vi "Teleop.vi"(10 "Match Info":T1={"Autonomous Elapsed Seconds"=0.0, "TeleOp Elapsed Seconds"=0.0, "Disabled Elapsed Seconds"=0.0, "Visited Autonomous"=FALSE, "Visited TeleOp"=FALSE, "Visited Disabled"=FALSE, "Autonomous Settings"={"Autonomous Style"=enum."Independent", "VI Refnum"=refnum}}, 11 "Call Context":T2) -> ()   [LabVIEW 2017]
doc: "This VI is called for each TeleOp packet received from the DS where the robot is not disabled. It is often used to read from the joysticks and update I/O or to update setpoints for timed control loops. It should complete and return within 20 milliseconds or it may miss DS packets."
uses:
  <vilib>/Rock Robotics/WPI/DriverStation/WPI_DriverStationDerivedRobotMode.ctl
  <vilib>/Rock Robotics/WPI/DriverStation/WPI_DriverStationMatch Info.ctl
  <vilib>/Rock Robotics/WPI/Utilities/WPI_GetSetVariantRefNum.vi
  <vilib>/Rock Robotics/WPI/RobotDrive/WPI_RobotDriveArcadeDrive_Standard(NoSaturation).vi
  Global Variables.vi
  <vilib>/Rock Robotics/Network Tables/NT Write Boolean Array.vi
  <vilib>/Rock Robotics/Network Tables/NT Write Numeric Array.vi
  <vilib>/Rock Robotics/Network Tables/NT Read Boolean.vi
  <vilib>/Rock Robotics/Network Tables/NT Read Number.vi
  <vilib>/Rock Robotics/WPI/RobotDrive/WPI_RobotDriveMecanumDrive_Cartesian.vi
panel:
  out "Sample Slider 0":dbl(slide) scale=0.0..5.0
  out "Sample Boolean 1":bool
  out "Sample Boolean 0":bool
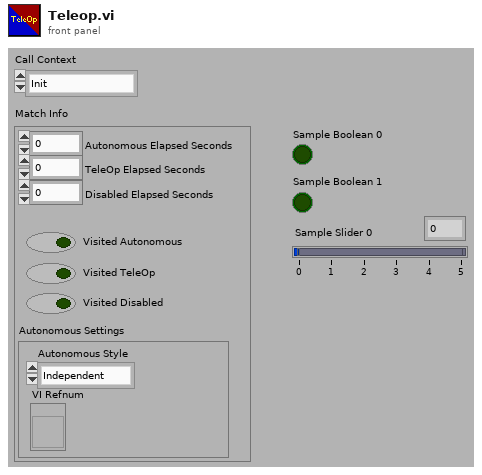
[diagram p1: front panel]
types:
  T1 = typedef "WPI_DriverStationMatch Info.ctl" = cluster{"Autonomous Elapsed Seconds":dbl, "TeleOp Elapsed Seconds":dbl, "Disabled Elapsed Seconds":dbl, "Visited Autonomous":bool, "Visited TeleOp":bool, "Visited Disabled":bool, "Autonomous Settings":cluster{"Autonomous Style":enum16{"Iterative", "Independent"}, "VI Refnum":refnum<vi>}}
  T2 = typedef "WPI_DriverStationDerivedRobotMode.ctl" = enum16{"Init", "Execute", "Stop"}
  T3 = typedef "WPI_RobotDriveDevRef.ctl" = cluster{"DevStatus":errorcluster, "Motors[]":T4[], "Square Inputs":bool, "Max Output":dbl}
  T4 = typedef "WPI_MotorControlDeviceRef.ctl" = cluster{"DeviceStatus":errorcluster, "Type":T5, "PWM":cluster{"PWM Channel":T6, "DeadBand":T7}, "CAN":cluster{"Device Number":u8, "SetOutput VI Ref":variant, "GetOutput VI Ref":variant, "Enable VI Ref":variant, "Disable VI Ref":variant, "Data":variant}, "Invert":bool, "DIO PWM":cluster{"PWM \"Enable\" Channel":T6, "DIOChannel":T8, "PWM Rate":dbl}}
  T5 = typedef "WPI_MotorControlType.ctl" = enum16{"PWM", "CAN", "DIO PWM"}
  T6 = typedef "FPGA_DIOPWMChannel.ctl" = enum8{"PWM 0", "PWM 1", "PWM 2", "PWM 3", "PWM 4", "PWM 5", "PWM 6", "PWM 7", "PWM 8", "PWM 9", "PWM MXP 0", "PWM MXP 1", "PWM MXP 2", "PWM MXP 3", "PWM MXP 4", "PWM MXP 5", "PWM MXP 6", "PWM MXP 7", "PWM MXP 8", "PWM MXP 9", "Invalid"}
  T7 = typedef "WPI_PWMDeadband.ctl" = cluster{"Name":string, "maxPositivePwm":i32, "minPositivePwm":i32, "centerPwm":i32, "maxNegativePwm":i32, "minNegativePwm":i32, "angularRange":u16}
  T8 = typedef "FPGA_DIOChannel.ctl" = enum8{"DIO 0", "DIO 1", "DIO 2", "DIO 3", "DIO 4", "DIO 5", "DIO 6", "DIO 7", "DIO 8", "DIO 9", "DIO MXP 0", "DIO MXP 1", "DIO MXP 2", "DIO MXP 3", "DIO MXP 4", "DIO MXP 5", "DIO MXP 6", "DIO MXP 7", "DIO MXP 8", "DIO MXP 9", "DIO MXP 10", "DIO MXP 11", "DIO MXP 12", "DIO MXP 13", "DIO MXP 14", "DIO MXP 15", "SPI Port CS1", "SPI Port CS2", "SPI Port CS3", "SPI Port MISO", "SPI Port MOSI", "Invalid"}
  T9 = typedef "WPI_JoystickDevRef.ctl" = cluster{"Device":T10}
  T10 = typedef "WPI_JoystickDeviceEnum.ctl" = enum16{"USB 0", "USB 1", "USB 2", "USB 3", "USB 4", "USB 5"}
  T11 = typedef "WPI_GyroDevRef.ctl" = cluster{"DevStatus":errorcluster, "Analog Channel":T12, "Gain (VoltsPerDegree/Second)":dbl, "Gyro Type":enum16{"Analog", "XRS450"}, "Handle":i32, "SPI Bus":T13, "Device Found":bool, "Sample Rate":dbl, "Calibrate On Open":bool, "Offset":dbl}
  T12 = typedef "FPGA_AIChannel.ctl" = enum8{"AI 0", "AI 1", "AI 2", "AI 3", "AI MXP 0", "AI MXP 1", "AI MXP 2", "AI MXP 3", "Invalid"}
  T13 = typedef "spi_bus.ctl" = enum16{"SPI On-Board, CS0", "SPI On-Board, CS1", "SPI On-Board, CS2", "SPI On-Board, CS3", "SPI MXP", "Invalid"}
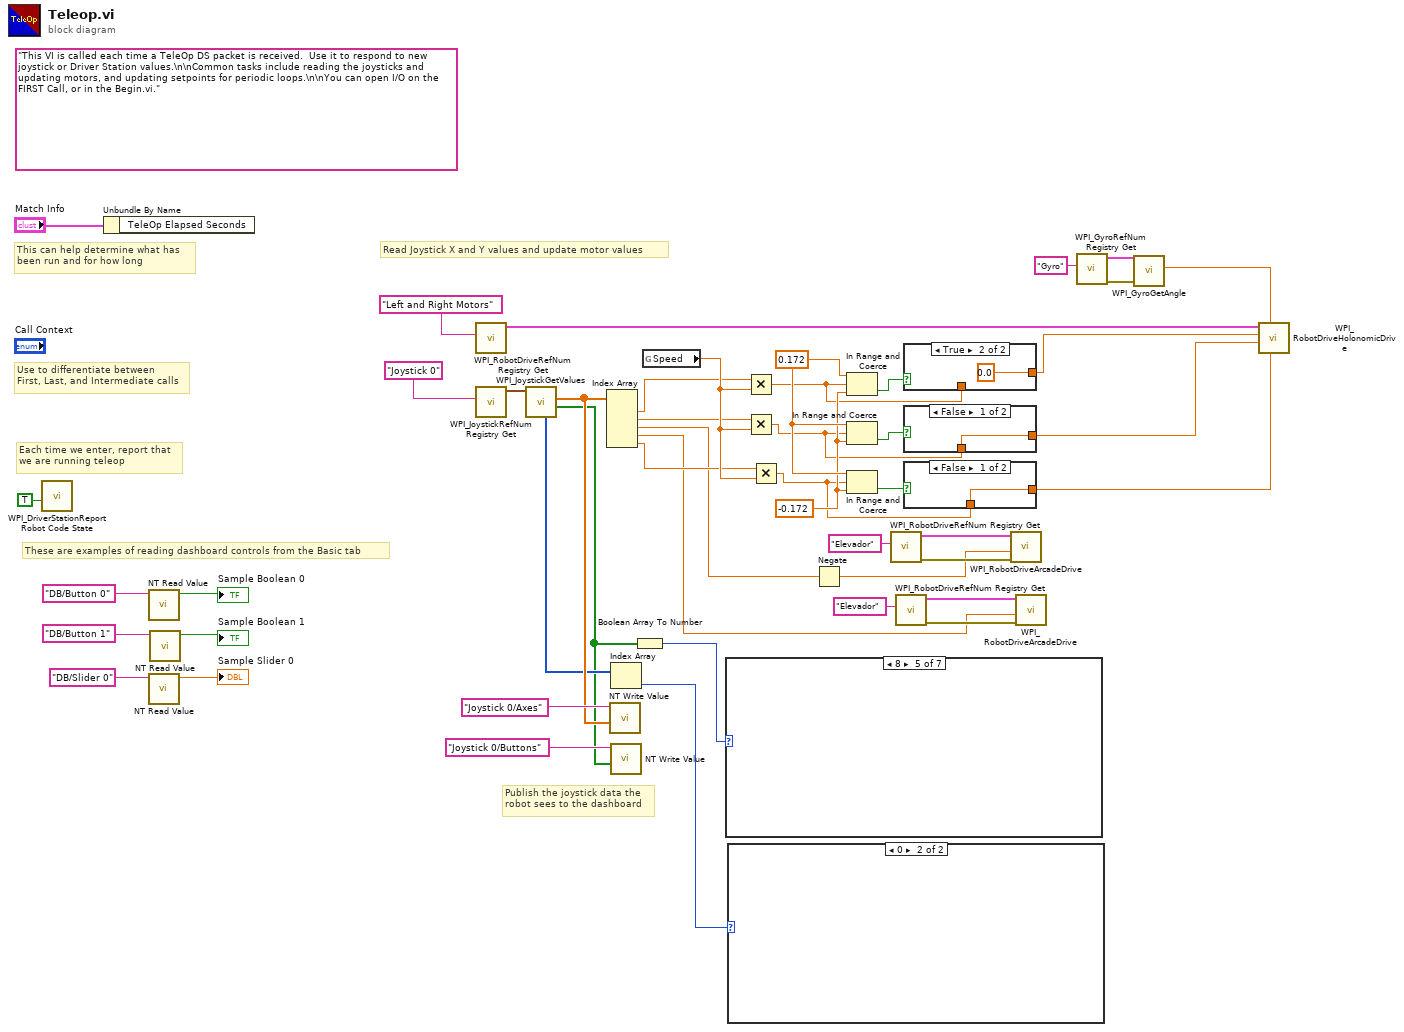
[diagram p0: block diagram]
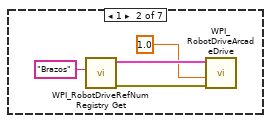
[diagram p4: hidden frame]
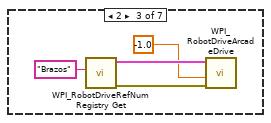
[diagram p5: hidden frame]
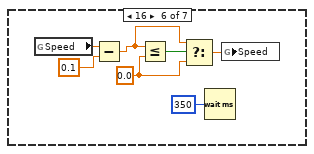
[diagram p7: hidden frame]
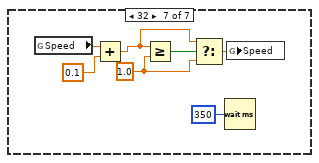
[diagram p8: hidden frame]
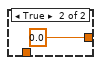
[diagram p9: hidden frame]
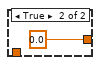
[diagram p10: hidden frame]
diagram:
  w33 = 0.172 ("lower limit")
  w32 = -0.172 ("lower limit")
  (unwired) "This VI is called each time a TeleOp DS packet is received.  Use it to respond to new joystick or Driver Station values.\n\nCommon tasks include reading the joysticks and updating motors, and updating setpoints for periodic loops.\n\nYou can open I/O on the FIRST Call, or in the Begin.vi."
  # "These are examples of reading dashboard controls from the Basic tab"
  # "Publish the joystick data the\nrobot sees to the dashboard"
  # "Each time we enter, report that\nwe are running teleop"
  # "Use to differentiate between\nFirst, Last, and Intermediate calls"
  # "This can help determine what has\nbeen run and for how long"
  # "Read Joystick X and Y values and update motor values"
  n1 = call <vilib>:"WPI_DriverStationReport Robot Code State.vi"("TeleOp"=TRUE ("Autonomous")) -> ()  [unwired: 10 in, 1 out]
  n2 = Unbundle By Name("Match Info") -> ()  [unwired: 1 out]
  n3 = call-poly <vilib>:"NT Read Value.vi"("Name"="DB/Button 0" ("refnum name")) -> ("Boolean"=→"Sample Boolean 0":bool)  [unwired: 9 in, 1 out]
  n4 = call-poly <vilib>:"NT Read Value.vi"("Name"="DB/Slider 0" ("refnum name")) -> ("Numeric"=→"Sample Slider 0":dbl)  [unwired: 9 in, 1 out]
  n5 = call-poly <vilib>:"NT Read Value.vi"("Name"="DB/Button 1" ("refnum name")) -> ("Boolean"=→"Sample Boolean 1":bool)  [unwired: 9 in, 1 out]
  n6 = call <vilib>:"WPI_RobotDriveRefNum Registry Get.vi"("refnum name"="Left and Right Motors") -> ("RobotDriveDevRef"=w25:T3)  [unwired: 1 in, 9 out]
  n7 = call <vilib>:"WPI_JoystickRefNum Registry Get.vi"("refnum name"="Joystick 0") -> ("JoystickDevRef"=w44:T9)  [unwired: 1 in, 9 out]
  n8 = call <vilib>:"WPI_JoystickGetValues.vi"("JoystickDevRef"=w44) -> ("Buttons"=w21:bool[], "Axes"=w40:dbl[], "POVs"=w23:i16[])  [unwired: 6 in, 2 out]
  n9 = Index Array(array=w40) -> (element #1=w19:dbl, element #2=w18:dbl, element #3=w2:dbl, element #4=w1:dbl, element #5=w14:dbl)  [unwired: 5 in]
  n10 = call-poly <vilib>:"NT Write Value.vi"("Numeric Array"=w40, "Name"="Joystick 0/Axes") -> ()  [unwired: 9 in, 1 out]
  n11 = Index Array(array=w23) -> (element=w22:i16)  [unwired: 1 in]
  n12 = call-poly <vilib>:"NT Write Value.vi"("Boolean Array"=w21, "Name"="Joystick 0/Buttons") -> ()  [unwired: 9 in, 1 out]
  n13 = Boolean Array To Number(Boolean array=w21) -> (number=w24:u32)
  n14 = global read "Global Variables.vi" "Speed"() -> (w20:dbl)
  n15 = case shown="8" w24 {
    frame 0, Default {
    }
    frame 1 {
      n16 = call <vilib>:"WPI_RobotDriveRefNum Registry Get.vi"("refnum name"="Brazos") -> ("error out"=w50:errorcluster, "RobotDriveDevRef"=w51:T3)  [unwired: 9 in]
      n17 = call-poly <vilib>:"WPI_RobotDriveArcadeDrive.vi"("error in (no error)"=w50, "Y axis value"=1.0, "RobotDriveDevRef"=w51) -> ()  [unwired: 6 in, 3 out]
    }
    frame 2 {
      n18 = call <vilib>:"WPI_RobotDriveRefNum Registry Get.vi"("refnum name"="Brazos") -> ("error out"=w54:errorcluster, "RobotDriveDevRef"=w55:T3)  [unwired: 9 in]
      n19 = call-poly <vilib>:"WPI_RobotDriveArcadeDrive.vi"("error in (no error)"=w54, "Y axis value"=-1.0, "RobotDriveDevRef"=w55) -> ()  [unwired: 6 in, 3 out]
    }
    frame 4 {
    }
    frame 8 {
    }
    frame 16 {
      w57 = 0.0 ("y")
      n20 = global read "Global Variables.vi" "Speed"() -> (w62:dbl)
      n21 = Subtract(x=w62, y=0.1) -> (x-y=w58:dbl)
      n22 = Less Or Equal?(x=w58, y=w57) -> (x <= y?=w60:bool)
      n23 = Select(t=w58, s=w60, f=w57) -> (s? t:f=w61:dbl)
      n24 = Wait (ms)(milliseconds to wait=u32 350) -> ()  [unwired: 1 out]
      n25 = global write "Global Variables.vi" "Speed"(w61) -> ()
    }
    frame 32 {
      w64 = 1.0 ("y")
      n26 = global read "Global Variables.vi" "Speed"() -> (w69:dbl)
      n27 = Add(x=w69, y=0.1) -> (x+y=w65:dbl)
      n28 = Greater Or Equal?(x=w65, y=w64) -> (x >= y?=w67:bool)
      n29 = Select(t=w65, s=w67, f=w64) -> (s? t:f=w68:dbl)
      n30 = Wait (ms)(milliseconds to wait=u32 350) -> ()  [unwired: 1 out]
      n31 = global write "Global Variables.vi" "Speed"(w68) -> ()
    }
  }
  n32 = case shown="0" w22 {
    frame -1, Default {
    }
    frame 0 {
    }
  }
  n33 = Multiply(x=w19, y=w20) -> (x*y=w16:dbl)
  n34 = Multiply(x=w18, y=w20) -> (x*y=w15:dbl)
  n35 = Multiply(x=w14, y=w20) -> (x*y=w17:dbl)
  n36 = Negate(x=w2) -> (-x=w3:dbl)
  n37 = In Range and Coerce(upper limit=w33, x=w16, lower limit=w32) -> (In Range?=w31:bool)  [unwired: 1 out]
  n38 = In Range and Coerce(upper limit=w33, x=w15, lower limit=w32) -> (In Range?=w30:bool)  [unwired: 1 out]
  n39 = In Range and Coerce(upper limit=w33, x=w17, lower limit=w32) -> (In Range?=w29:bool)  [unwired: 1 out]
  n40 = call <vilib>:"WPI_RobotDriveRefNum Registry Get.vi"("refnum name"="Elevador") -> ("error out"=w8:errorcluster, "RobotDriveDevRef"=w9:T3)  [unwired: 9 in]
  n41 = call <vilib>:"WPI_RobotDriveRefNum Registry Get.vi"("refnum name"="Elevador") -> ("error out"=w6:errorcluster, "RobotDriveDevRef"=w5:T3)  [unwired: 9 in]
  n42 = case shown="True" w31 {
    tunnel: [w70 0.0 ("upper limit")] -> w28
    tunnel: w16 -> [w70 _]
    frame False {
    }
    frame True {
    }
  }
  n43 = case shown="False" w30 {
    tunnel: [w72 0.0 ("upper limit")] -> w27
    tunnel: w15 -> [w72 _]
    frame False {
    }
    frame True {
    }
  }
  n44 = case shown="False" w29 {
    tunnel: [w74 0.0 ("upper limit")] -> w26
    tunnel: w17 -> [w74 _]
    frame False {
    }
    frame True {
    }
  }
  n45 = call-poly <vilib>:"WPI_RobotDriveArcadeDrive.vi"("error in (no error)"=w8, "Y axis value"=w3, "RobotDriveDevRef"=w9) -> ()  [unwired: 6 in, 3 out]
  n46 = call-poly <vilib>:"WPI_RobotDriveArcadeDrive.vi"("error in (no error)"=w6, "Y axis value"=w1, "RobotDriveDevRef"=w5) -> ()  [unwired: 6 in, 3 out]
  n47 = call <vilib>:"WPI_GyroRefNum Registry Get.vi"("refnum name"="Gyro") -> ("error out"=w13:errorcluster, "GyroDevRef"=w12:T11)  [unwired: 9 in]
  n48 = call <vilib>:"WPI_GyroGetAngle.vi"("error in"=w13, "GyroDevRef"=w12) -> ("Angle"=w11:dbl)  [unwired: 5 in, 4 out]
  n49 = call-poly <vilib>:"WPI_RobotDriveHolonomicDrive.vi"("Rotation"=w26, "Gyro Angle"=w11, "Y"=w27, "X"=w28, "RobotDriveDevRef"=w25) -> ()  [unwired: 4 in, 3 out]
